vi "ParseMarkerPacket.vi"(0 "Packet":string) -> (1 "Bytes":u32, 2 "MessageID":u32, 3 "FrameNum":u32, 4 "NumMarkerSets":u32, 6 "MarkerSets":T3(array[cluster]), 8 "UnIDMarkers":T2, 10 "NumRigidBodies":u32, 12 "Remaining":string, 14 "MarkerDataValid":bool, 15 "RigidBodies":T1(array[cluster]))   [LabVIEW 2011]
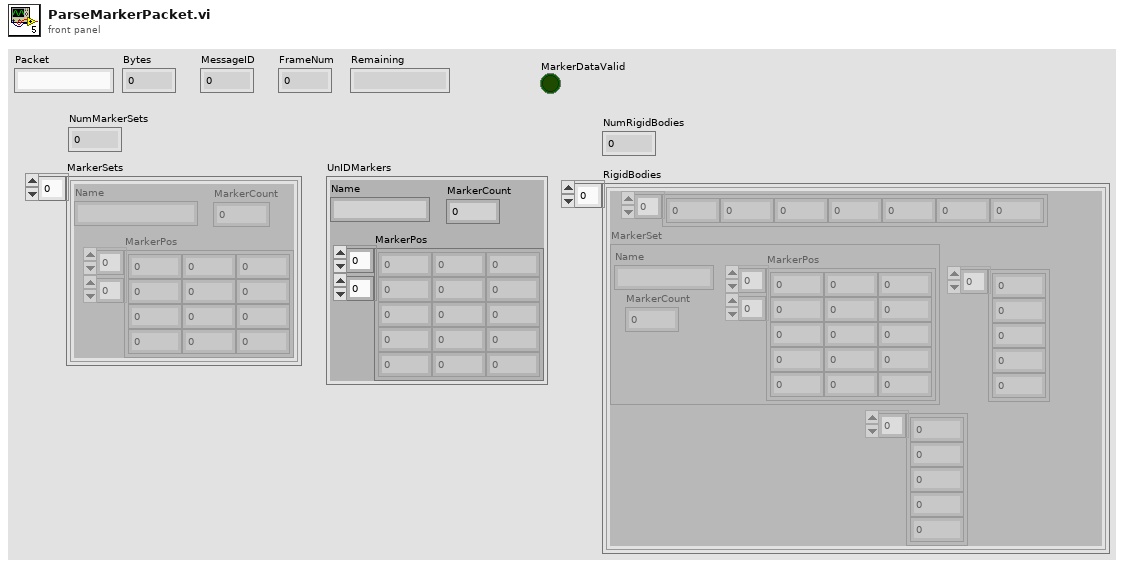
[diagram p1: front panel]
types:
  T1 = cluster{sgl[], "MarkerSet":cluster{"Name":string, "MarkerCount":u32, "MarkerPos":sgl[][]}, u32[], sgl[]}[]
  T2 = cluster{"Name":string, "MarkerCount":u32, "MarkerPos":sgl[][]}
  T3 = cluster{"Name":string, "MarkerCount":u32, "MarkerPos":sgl[][]}[]
  T4 = cluster{sgl[], "MarkerSet":cluster{"Name":string, "MarkerCount":u32, "MarkerPos":sgl[][]}, u32[], sgl[]}
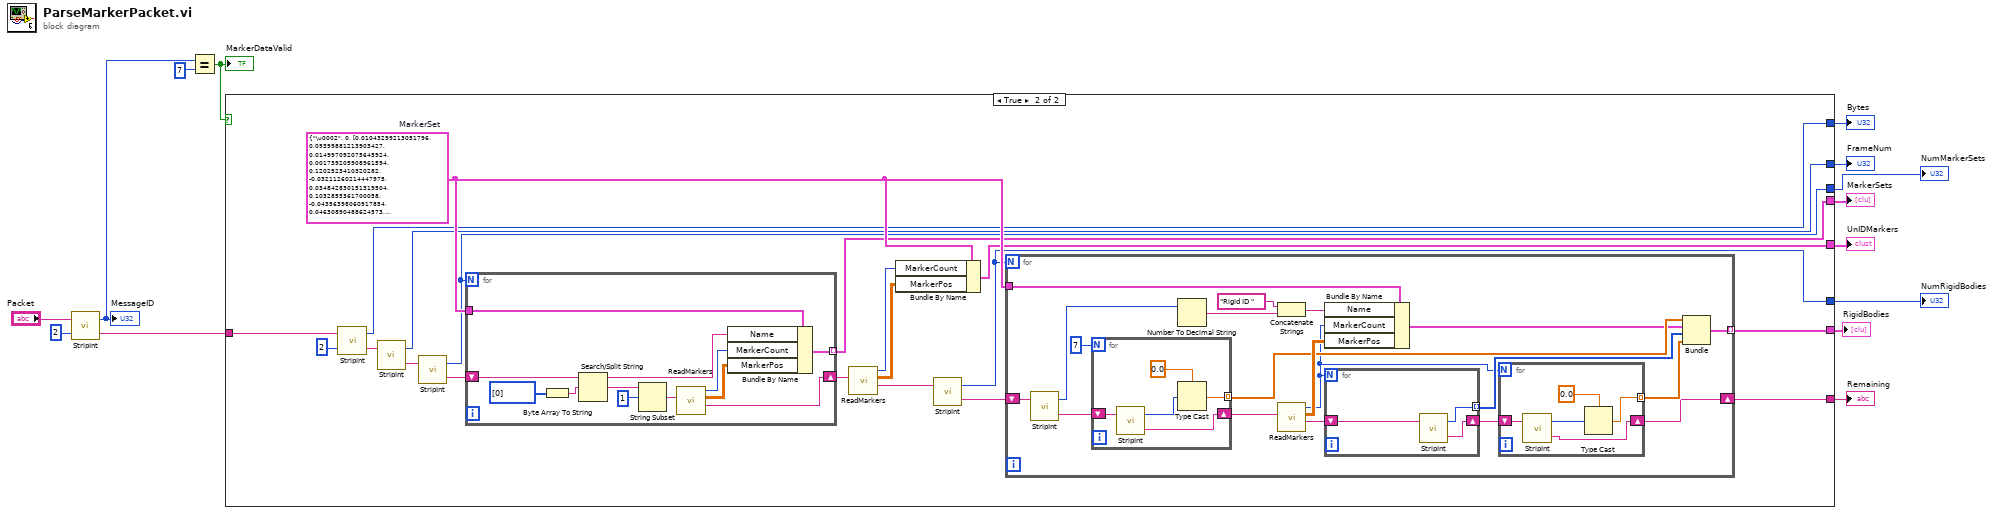
[diagram p0: block diagram]
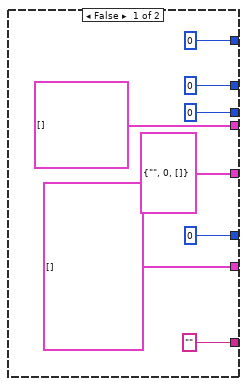
[diagram p2: hidden frame]
diagram:
  n1 = call "StripInt.vi"("Width"=2, "String"="Packet") -> ("Remaining"=w10:string, "Value"=w12:u32)
  "MessageID" <- w12
  n2 = Equal?(x=w12, y=u32 7) -> (x = y?=w14:bool)
  "MarkerDataValid" <- w14
  n3 = case shown="True" w14 {
    tunnel: w10 -> [_ w41]
    tunnel: ["" ("Remaining") w24] -> w11
    tunnel: [u32 0 ("Value") w30] -> w7
    tunnel: [T2 {"Name"="", "MarkerCount"=0, "MarkerPos"=[]} ("MarkerSet") w29] -> w6
    tunnel: [T3 [] w28] -> w5
    tunnel: [u32 0 ("Value") w27] -> w4
    tunnel: [u32 0 ("Value") w26] -> w3
    tunnel: [u32 0 ("Value") w25] -> w2
    tunnel: [T1 [] w23] -> w1
    frame False {
    }
    frame True {
      w31 = T2 {"Name"="\u0002", "MarkerCount"=0, "MarkerPos"=[[0.010432992, 0.09399881, 0.014997092], [0.0017392059, 0.12025234, -0.032112602], [0.03484283, 0.103285536, -0.04356398], [0.046308905, 0.090583004, 0.0047033187]]}  # MarkerSet
      n4 = call "StripInt.vi"("Width"=2, "String"=w41) -> ("Remaining"=w39:string, "Value"=w25:u32)
      n5 = call "StripInt.vi"("String"=w39) -> ("Remaining"=w38:string, "Value"=w26:u32)  [unwired: 1 in]
      n6 = call "StripInt.vi"("String"=w38) -> ("Remaining"=w37:string, "Value"=w27:u32)  [unwired: 1 in]
      n7 = for {
        N: w27 -> [_]
        shift-right: [w80] -> w36
        shift-left: w37 -> [w76]
        tunnel: [w75] -> w28 mode=indexing
        tunnel: w31 -> [w74]
        n8 = Byte Array To String(unsigned byte array=u8[] [0]) -> (string=w84:string)
        n9 = Search/Split String(string=w76, search string/char (-)=w84) -> (substring before match=w79:string, match + rest of string=w83:string)  [unwired: 1 in, 1 out]
        n10 = String Subset(string=w83, offset (0)=1) -> (substring=w81:string)  [unwired: 1 in]
        n11 = call "ReadMarkers.vi"("Data"=w81) -> ("Remaining"=w80:string, "Markers"=w77:sgl[][], "MarkerCount"=w78:u32)  [unwired: 8 in]
        n12 = Bundle By Name(cluster=w74, "Name"=w79, "MarkerCount"=w78, "MarkerPos"=w77) -> (w75:T2)
      }
      n13 = call "ReadMarkers.vi"("Data"=w36) -> ("Remaining"=w33:string, "Markers"=w34:sgl[][], "MarkerCount"=w35:u32)  [unwired: 8 in]
      n14 = Bundle By Name(cluster=w31, "MarkerCount"=w35, "MarkerPos"=w34) -> (w29:T2)
      n15 = call "StripInt.vi"("String"=w33) -> ("Remaining"=w32:string, "Value"=w30:u32)  [unwired: 1 in]
      n16 = for {
        N: w30 -> [_]
        shift-right: [w42] -> w24
        shift-left: w32 -> [w58]
        tunnel: w31 -> [w59]
        tunnel: [w43] -> w23 mode=indexing
        n17 = call "StripInt.vi"("String"=w58) -> ("Remaining"=w53:string, "Value"=w57:u32)  [unwired: 1 in]
        n18 = for {
          N: 7 ("Elements") -> [_]
          shift-right: [w72] -> w52
          shift-left: w53 -> [w73]
          tunnel: [w70] -> w51 mode=indexing
          n19 = call "StripInt.vi"("String"=w73) -> ("Remaining"=w72:string, "Value"=w71:u32)  [unwired: 1 in]
          n20 = Type Cast(type=sgl 0.0, x=w71) -> (*(type *) &x=w70:sgl)
        }
        n21 = Number To Decimal String(number=w57) -> (decimal integer string=w56:string)  [unwired: 1 in]
        n22 = Concatenate Strings("Rigid ID " ("string"), w56) -> (w49:string)
        n23 = call "ReadMarkers.vi"("Data"=w52) -> ("Remaining"=w48:string, "Markers"=w60:sgl[][], "MarkerCount"=w45:u32)  [unwired: 8 in]
        n24 = Bundle By Name(cluster=w59, "Name"=w49, "MarkerCount"=w45, "MarkerPos"=w60) -> (w50:T2)
        n25 = for {
          N: w45 -> [_]
          shift-right: [w67] -> w46
          shift-left: w48 -> [w68]
          tunnel: [w66] -> w47 mode=indexing
          n26 = call "StripInt.vi"("String"=w68) -> ("Remaining"=w67:string, "Value"=w66:u32)  [unwired: 1 in]
        }
        n27 = for {
          N: w45 -> [_]
          shift-right: [w64] -> w42
          shift-left: w46 -> [w65]
          tunnel: [w61] -> w44 mode=indexing
          n28 = call "StripInt.vi"("String"=w65) -> ("Remaining"=w64:string, "Value"=w62:u32)  [unwired: 1 in]
          n29 = Type Cast(type=sgl 0.0, x=w62) -> (*(type *) &x=w61:sgl)
        }
        n30 = Bundle(w51, "MarkerSet"=w50, w47, w44) -> (w43:T4)  [unwired: 1 in]
      }
    }
  }
  "Remaining" <- w11
  "NumRigidBodies" <- w7
  "UnIDMarkers" <- w6
  "MarkerSets" <- w5
  "NumMarkerSets" <- w4
  "FrameNum" <- w3
  "Bytes" <- w2
  "RigidBodies" <- w1
